vi "Uni-string-read_HistogramArray.vi"(9 "error in":errorcluster, 10 "file (use dialog)":path) -> (1 "error out":errorcluster, 2 "output string":string, 3 "Histogram Array":dbl[][](array[numeric]), 4 "UTF-8":bool, 5 "special characters detected":bool, 6 "unicode-bigendian":bool, 7 "unicode":bool)   [LabVIEW 2018]
panel:
  out "unsigned byte array":u8[](array[numeric])
  # "This module is designed to read unicode text files that contain plan text without special characters.\n\nIf a string is unicode, converts it to plain text, otherwise leaves it unchanged.  There is provision for dealing with special characters, but at the moment they are only flagged in unicode and unicode-bigendian.  UTF-7 and UTF-8 special characters are not detected.\n\nEnhancements welcome.\nJames.Trevelyan@uwa.edu.au"
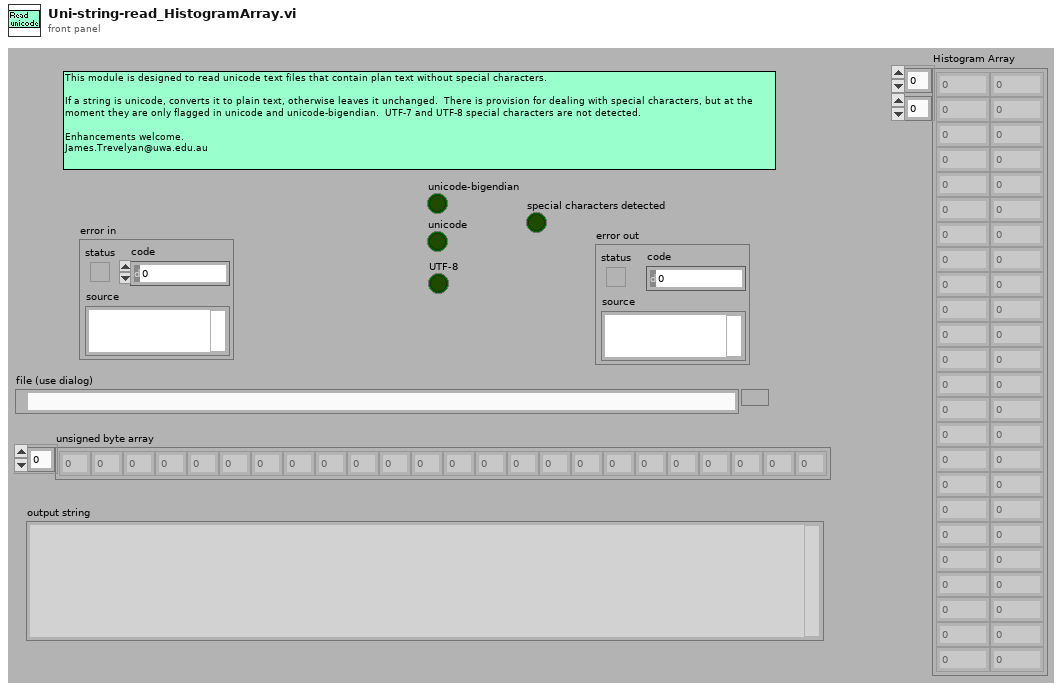
[diagram p1: front panel]
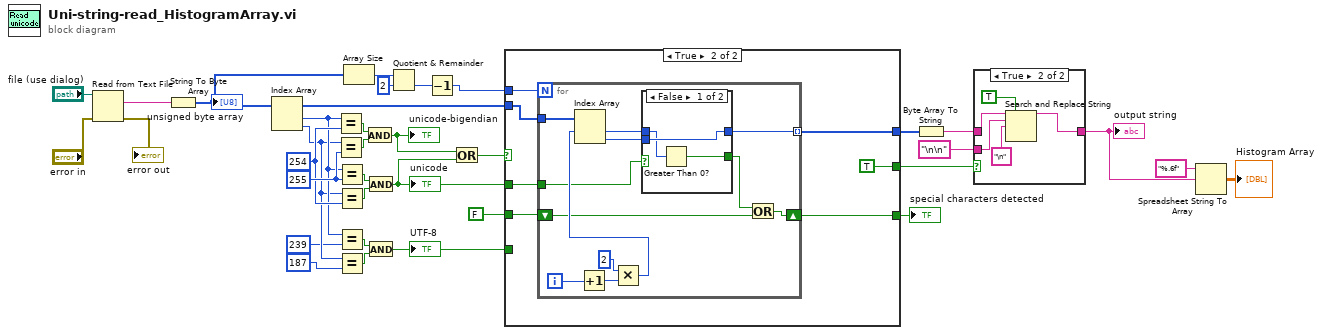
[diagram p0: block diagram]
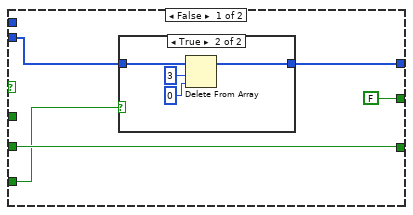
[diagram p3: hidden frame]
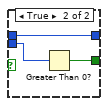
[diagram p5: hidden frame]
diagram:
  w31 = u8 254 ("y")
  w32 = u8 255 ("y")
  n1 = Read from Text File(file (use dialog)="file (use dialog)", error in="error in") -> (text=w33:string, error out=→"error out":errorcluster)  [unwired: 2 in, 2 out]
  n2 = String To Byte Array(string=w33) -> (unsigned byte array=w22:u8[])
  "unsigned byte array" <- w22
  n3 = Index Array(array=w22) -> (element #1=w13:u8, element #2=w12:u8)  [unwired: 2 in]
  n4 = Equal?(x=w13, y=w31) -> (x = y?=w29:bool)
  n5 = Equal?(x=w12, y=w32) -> (x = y?=w30:bool)
  n6 = Equal?(x=w13, y=w32) -> (x = y?=w28:bool)
  n7 = Equal?(x=w12, y=w31) -> (x = y?=w27:bool)
  n8 = Equal?(x=w13, y=u8 239) -> (x = y?=w14:bool)
  n9 = Equal?(x=w12, y=u8 187) -> (x = y?=w15:bool)
  n10 = Array Size(array=w22) -> (size(s)=w26:i32)
  n11 = And(x=w29, y=w30) -> (x .and. y?=w23:bool)
  "unicode-bigendian" <- w23
  n12 = And(x=w28, y=w27) -> (x .and. y?=w21:bool)
  "unicode" <- w21
  n13 = And(x=w14, y=w15) -> (x .and. y?=w9:bool)
  "UTF-8" <- w9
  n14 = Quotient & Remainder(x=w26, y=2) -> (floor(x/y)=w17:i32)  [unwired: 1 out]
  n15 = Decrement(x=w17) -> (x-1=w16:i32)
  n16 = Or(x=w23, y=w21) -> (x .or. y?=w24:bool)
  n17 = case shown="True" w24 {
    tunnel: w16 -> [_ w51]
    tunnel: w22 -> [w38 w50]
    tunnel: w21 -> [_ w49]
    tunnel: FALSE -> [w39 w48]
    tunnel: [w36 w47] -> w19
    tunnel: [w39 w46] -> w18
    tunnel: w9 -> [w37 _]
    tunnel: [FALSE TRUE] -> w7
    frame False {
      n18 = case shown="True" w37 {
        tunnel: w38 -> [w40 w44]
        tunnel: [w40 w43] -> w36
        frame False {
        }
        frame True {
          n19 = Delete From Array(array=w44, length=3, index=0) -> (array with subset deleted=w43:u8[])  [unwired: 1 out]
        }
      }
    }
    frame True {
      n20 = for {
        N: w51 -> [_]
        tunnel: w50 -> [w62]
        tunnel: w49 -> [w60]
        shift-right: [w55] -> w46
        shift-left: w48 -> [w57]
        tunnel: [w54] -> w47 mode=indexing
        i -> [w53]
        n21 = Increment(x=w53) -> (x+1=w52:i32)
        n22 = Multiply(x=2, y=w52) -> (x*y=w61:i32)
        n23 = Index Array(array=w62, index #1=w61) -> (element #1=w59:u8, element #2=w58:u8)  [unwired: 1 in]
        n24 = case shown="False" w60 {
          tunnel: w59 -> [w65 w69]
          tunnel: w58 -> [w66 w67]
          tunnel: [w66 w69] -> w54
          tunnel: [w64 w68] -> w56
          frame False {
            n25 = Greater Than 0?(x=w65) -> (x > 0?=w64:bool)
          }
          frame True {
            n26 = Greater Than 0?(x=w67) -> (x > 0?=w68:bool)
          }
        }
        n27 = Or(x=w56, y=w57) -> (x .or. y?=w55:bool)
      }
    }
  }
  "special characters detected" <- w18
  n28 = Byte Array To String(unsigned byte array=w19) -> (string=w8:string)
  n29 = case shown="True" w7 {
    tunnel: w8 -> [w70 w75]
    tunnel: [w70 w74] -> w3
    tunnel: "\n\n" -> [_ w73]
    frame False {
    }
    frame True {
      n30 = Search and Replace String(replace all?=TRUE ("replace all? (F)"), input string=w75, search string=w73, replace string="\n") -> (result string=w74:string)  [unwired: 4 in, 3 out]
    }
  }
  "output string" <- w3
  n31 = Spreadsheet String To Array(format string="%.6f", spreadsheet string=w3) -> (array=→"Histogram Array":dbl[][])  [unwired: 2 in]
